vi "GetCtrlPanelRef.vi"(2 "error in (no error)":errorcluster, 3 "Ctrl Refnum":refnum<vi>) -> (0 "error out":errorcluster, 1 "Ctrl Panel Ref":refnum<vi>)   [LabVIEW 2013]
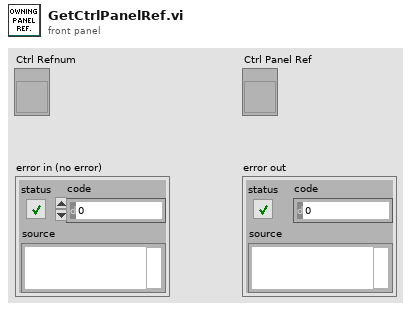
[diagram p1: front panel]
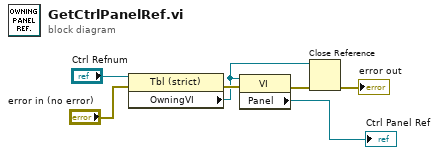
[diagram p0: block diagram]
diagram:
  n1 = property class="Tbl (strict)"(reference="Ctrl Refnum", error in="error in (no error)") -> (error out=w5:errorcluster, "OwningVI"=w1:refnum<vi>)  [unwired: 1 out]
  n2 = property class="VI"(reference=w1, error in=w5) -> (error out=w3:errorcluster, "Panel"=→"Ctrl Panel Ref":refnum<vi>)  [unwired: 1 out]
  n3 = Close Reference(reference=w1, error in (no error)=w3) -> (error out=→"error out":errorcluster)
